vi "Average_Data.vi"(0 "Data in":dbl[](array[numeric])) -> (1 "Average DBL":dbl, 2 "Average U32":u32)   [LabVIEW 2017]
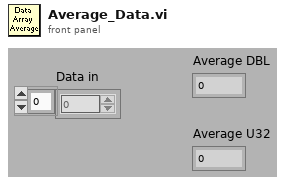
[diagram p1: front panel]
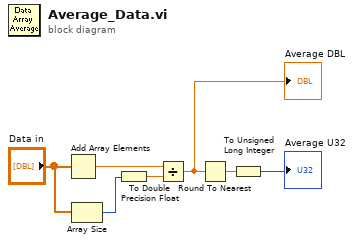
[diagram p0: block diagram]
diagram:
  n1 = Add Array Elements(numeric array="Data in") -> (sum=w6:dbl)
  n2 = Array Size(array="Data in") -> (size(s)=w5:i32)
  n3 = To Double Precision Float(number=w5) -> (double precision float=w4:dbl)
  n4 = Divide(x=w6, y=w4) -> (x/y=w3:dbl)
  "Average DBL" <- w3
  n5 = Round To Nearest(number=w3) -> (nearest integer value=w2:dbl)
  n6 = To Unsigned Long Integer(number=w2) -> (unsigned 32bit integer=→"Average U32":u32)
